vi "Generic command handler.vi"(8 "error in (no error)":errorcluster, 10 "Message in":refnum<class "GenericMessage.lvclass">, 11 "DAQMH121119OrcaFlash in":refnum<class "DAQOrcaFlash.lvclass">) -> (0 "error out":errorcluster, 2 "value":string, 3 "DAQMH121119OrcaFlash out":refnum<class "DAQOrcaFlash.lvclass">)   [LabVIEW 2012, in "DAQOrcaFlash.lvclass"]
doc: "The generic_command_handler processes the command 'generic'. Commands which are not part of the predefined list of commands fall under the 'generic' command for special activity."
uses:
  DAQOrcaFlash.lvclass
  <vilib>/Distrio/Murmex/GenericMessage/GenericMessage.lvclass
  <vilib>/Distrio/Murmex/Murmex/Murmex.lvclass
  <vilib>/Distrio/Murmex/ProceedMessage/ProceedMessage.lvclass
  DAQOrcaFlash.lvclass/DAQOrcaFlash.ctl
  <vilib>/Distrio/Murmex/Message/Message.lvclass
  <vilib>/Distrio/Murmex/ResetMessage/ResetMessage.lvclass
panel:
  # "This method is called when the GENERIC\ntrigger is sent. \n\nOverride this method when your component needs to\nrespond to this trigger. \n\nCall parent for proper implementation"
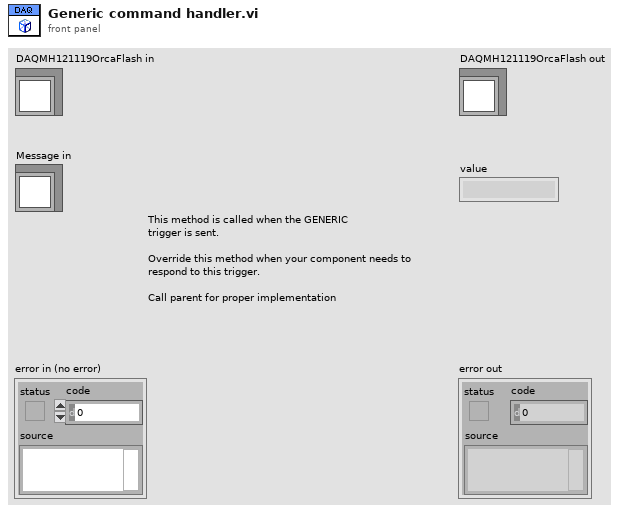
[diagram p1: front panel]
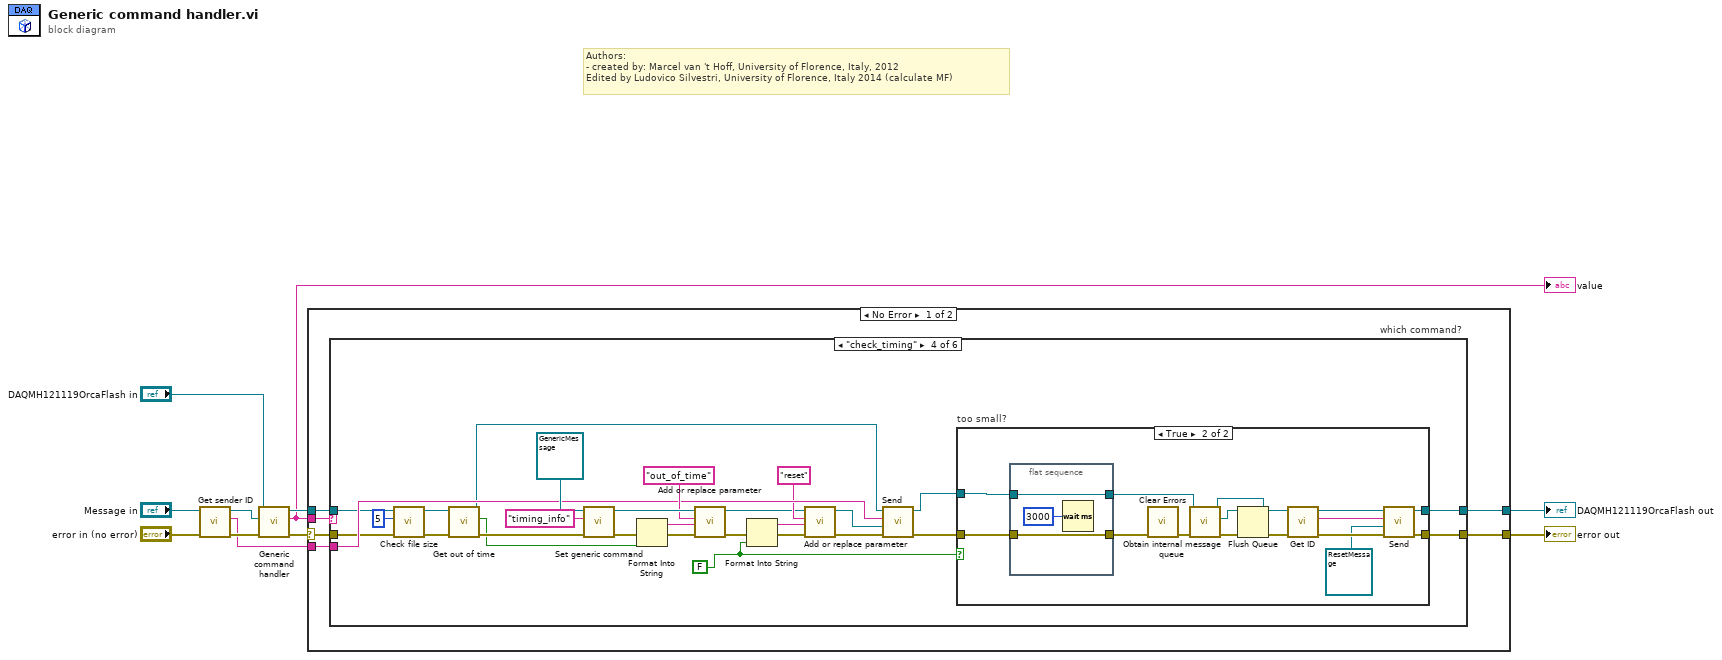
[diagram p0: block diagram]
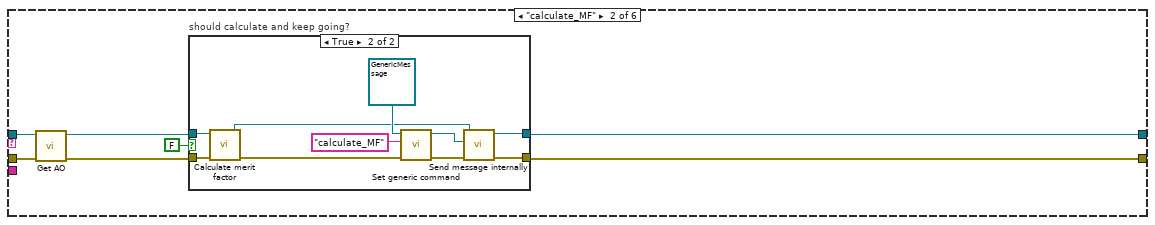
[diagram p3: hidden frame]
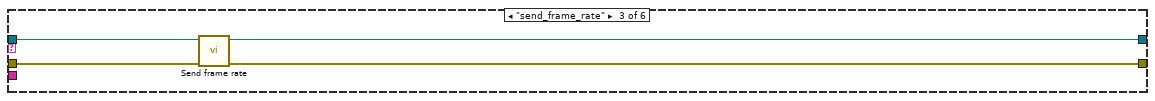
[diagram p5: hidden frame]
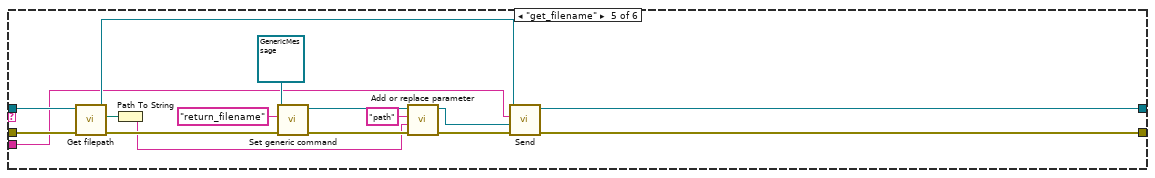
[diagram p7: hidden frame]
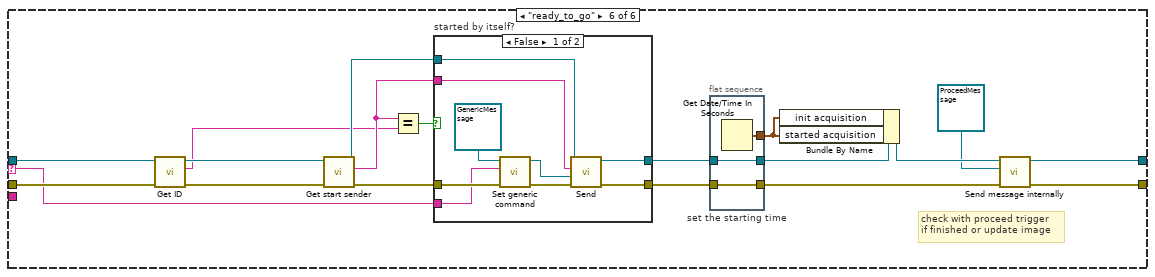
[diagram p8: hidden frame]
diagram:
  # "Authors: \n- created by: Marcel van 't Hoff, University of Florence, Italy, 2012\nEdited by Ludovico Silvestri, University of Florence, Italy 2014 (calculate MF)"
  n1 = call <vilib>:"Get sender ID.vi"("error in (no error)"="error in (no error)", "Message in"="Message in") -> ("error out"=w4:errorcluster, "sender"=w1:string, "Message out"=w2:refnum<class "GenericMessage.lvclass">)  [unwired: 7 in]
  n2 = call-parent "Generic command handler.vi"("error in (no error)"=w4, "Message in"=w2, "Murmex in"="DAQMH121119OrcaFlash in") -> ("error out"=w9:errorcluster, "value"=w5:string, "Murmex out"=w6:refnum<class "DAQOrcaFlash.lvclass">)  [unwired: 6 in]
  "value" <- w5
  n3 = case shown="No Error" w9 {
    selector: w9 -> [w16 w141]
    tunnel: [w15 w141] -> w8
    tunnel: [w14 w140] -> w7
    tunnel: w6 -> [w13 w140]
    tunnel: w5 -> [w17 _]
    tunnel: w1 -> [w12 _]
    frame No Error {
      n4 = case "which command?" shown="\"check_timing\"" w17 {
        selector: w17 -> [_ _ _ _ _ w123]
        tunnel: w16 -> [w19 w26 w42 w57 w105 w125]
        tunnel: w13 -> [w18 w25 w41 w59 w106 w120]
        tunnel: [w19 w22 w40 w44 w91 w110] -> w15
        tunnel: [w18 w21 w39 w45 w92 w108] -> w14
        tunnel: w12 -> [_ _ _ w63 w94 _]
        frame Default {
        }
        frame "calculate_MF" {
          n5 = call-dynamic "Get AO.vi"("error in (no error)"=w26, "DAQOrcaFlash in"=w25) -> ("error out"=w24:errorcluster, "DAQOrcaFlash out"=w23:refnum<class "DAQOrcaFlash.lvclass">)  [unwired: 7 in, 1 out]
          n6 = case "should calculate and keep going?" shown="True" FALSE {
            tunnel: w24 -> [w28 w38]
            tunnel: w23 -> [w27 w37]
            tunnel: [w28 w32] -> w22
            tunnel: [w27 w34] -> w21
            frame False {
            }
            frame True {
              n7 = call-dynamic "Calculate merit factor.vi"("error in (no error)"=w38, "DAQOrcaFlash in"=w37) -> ("error out"=w29:errorcluster, "DAQOrcaFlash out"=w30:refnum<class "DAQOrcaFlash.lvclass">)  [unwired: 8 in]
              n8 = call <vilib>:"Set generic command.vi"("error in (no error)"=w29, "generic command"="calculate_MF", "GenericMessage in"=refnum<class "GenericMessage.lvclass"> refnum ("GenericMessage")) -> ("error out"=w33:errorcluster, "GenericMessage out"=w31:refnum<class "GenericMessage.lvclass">)  [unwired: 7 in]
              n9 = call <vilib>:"Send message internally.vi"("error in (no error)"=w33, "Message"=w31, "Murmex in"=w30) -> ("error out"=w32:errorcluster, "Murmex out"=w34:refnum<class "DAQOrcaFlash.lvclass">)  [unwired: 7 in]
            }
          }
        }
        frame "send_frame_rate" {
          n10 = call-dynamic "Send frame rate.vi"("error in (no error)"=w42, "DAQOrcaFlash in"=w41) -> ("error out"=w40:errorcluster, "DAQOrcaFlash out"=w39:refnum<class "DAQOrcaFlash.lvclass">)  [unwired: 8 in]
        }
        frame "check_timing" {
          w43 = FALSE
          n11 = call-dynamic "Check file size.vi"("error in (no error)"=w57, "min size (KB)"=i64 5, "DAQOrcaFlash in"=w59) -> ("error out"=w56:errorcluster, "DAQOrcaFlash out"=w58:refnum<class "DAQOrcaFlash.lvclass">)  [unwired: 6 in, 1 out]
          n12 = call-dynamic "Get out of time.vi"("error in (no error)"=w56, "DAQOrcaFlash in"=w58) -> ("error out"=w62:errorcluster, "out of time?"=w60:bool, "DAQOrcaFlash out"=w61:refnum<class "DAQOrcaFlash.lvclass">)  [unwired: 7 in]
          n13 = call <vilib>:"Set generic command.vi"("error in (no error)"=w62, "generic command"="timing_info", "GenericMessage in"=refnum<class "GenericMessage.lvclass"> refnum ("Distrio Murmex 1.5:GenericMessage")) -> ("error out"=w66:errorcluster, "GenericMessage out"=w68:refnum<class "GenericMessage.lvclass">)  [unwired: 7 in]
          n14 = Format Into String(error in=w66, w60) -> (resulting string=w64:string, error out=w65:errorcluster)  [unwired: 2 in]
          n15 = call <vilib>:"Add or replace parameter.vi"("error in (no error)"=w65, "value"=w64, "name"="out_of_time", "Message in"=w68) -> ("error out"=w51:errorcluster, "Message out"=w49:refnum<class "GenericMessage.lvclass">)  [unwired: 6 in]
          n16 = Format Into String(error in=w51, w43) -> (resulting string=w52:string, error out=w53:errorcluster)  [unwired: 2 in]
          n17 = call <vilib>:"Add or replace parameter.vi"("error in (no error)"=w53, "value"=w52, "name"="reset", "Message in"=w49) -> ("error out"=w50:errorcluster, "Message out"=w48:refnum<class "GenericMessage.lvclass">)  [unwired: 6 in]
          n18 = call <vilib>:"Send.vi"("error in (no error)"=w50, "Message"=w48, "recipient"=w63, "Murmex in"=w61) -> ("error out"=w46:errorcluster, "Murmex out"=w47:refnum<class "DAQOrcaFlash.lvclass">)  [unwired: 6 in]
          n19 = case "too small?" shown="True" w43 {
            tunnel: w46 -> [w72 w83]
            tunnel: w47 -> [w71 w81]
            tunnel: [w72 w79] -> w44
            tunnel: [w71 w75] -> w45
            frame False {
            }
            frame True {
              n20 = flat-sequence {
                tunnel: [w90] -> w84
                tunnel: w83 -> [w90]
                tunnel: [w89] -> w82
                tunnel: w81 -> [w89]
                frame #0 {
                  n21 = Wait (ms)(milliseconds to wait=u32 3000) -> ()  [unwired: 1 out]
                }
              }
              n22 = call <vilib>:"Clear Errors.vi"("error in (no error)"=w84) -> ("error out"=w87:errorcluster)  [unwired: 6 in]
              n23 = call <vilib>:"Obtain internal message queue.vi"("error in (no error)"=w87, "Murmex in"=w82) -> ("error out"=w85:errorcluster, "internal message queue"=w86:refnum<queue>, "Murmex out"=w77:refnum<class "DAQOrcaFlash.lvclass">)  [unwired: 7 in]
              n24 = Flush Queue(queue=w86, error in (no error)=w85) -> (error out=w78:errorcluster)  [unwired: 2 out]
              n25 = call <vilib>:"Get ID.vi"("error in (no error)"=w78, "Murmex in"=w77) -> ("error out"=w80:errorcluster, "component id"=w74:string, "Murmex out"=w76:refnum<class "DAQOrcaFlash.lvclass">)  [unwired: 7 in]
              n26 = call <vilib>:"Send.vi"("error in (no error)"=w80, "Message"=refnum<class "ResetMessage.lvclass"> refnum ("Message in"), "recipient"=w74, "Murmex in"=w76) -> ("error out"=w79:errorcluster, "Murmex out"=w75:refnum<class "DAQOrcaFlash.lvclass">)  [unwired: 6 in]
            }
          }
        }
        frame "get_filename" {
          n27 = call "Get filepath.vi"("error in (no error)"=w105, "DAQOrcaFlash in"=w106) -> ("error out"=w102:errorcluster, "full storage path"=w98:path, "DAQOrcaFlash out"=w95:refnum<class "DAQOrcaFlash.lvclass">)  [unwired: 7 in]
          n28 = Path To String(path=w98) -> (string=w97:string)
          n29 = call <vilib>:"Set generic command.vi"("error in (no error)"=w102, "generic command"="return_filename", "GenericMessage in"=refnum<class "GenericMessage.lvclass"> refnum ("Message in")) -> ("error out"=w101:errorcluster, "GenericMessage out"=w100:refnum<class "GenericMessage.lvclass">)  [unwired: 7 in]
          n30 = call <vilib>:"Add or replace parameter.vi"("error in (no error)"=w101, "value"=w97, "name"="path", "Message in"=w100) -> ("error out"=w96:errorcluster, "Message out"=w93:refnum<class "GenericMessage.lvclass">)  [unwired: 6 in]
          n31 = call <vilib>:"Send.vi"("error in (no error)"=w96, "Message"=w93, "recipient"=w94, "Murmex in"=w95) -> ("error out"=w91:errorcluster, "Murmex out"=w92:refnum<class "DAQOrcaFlash.lvclass">)  [unwired: 6 in]
        }
        frame "ready_to_go" {
          # "check with proceed trigger\nif finished or update image"
          n32 = call <vilib>:"Get ID.vi"("error in (no error)"=w125, "Murmex in"=w120) -> ("error out"=w121:errorcluster, "component id"=w116:string, "Murmex out"=w119:refnum<class "DAQOrcaFlash.lvclass">)  [unwired: 7 in]
          n33 = call-dynamic "Get start sender.vi"("error in (no error)"=w121, "DAQOrcaFlash in"=w119) -> ("error out"=w124:errorcluster, "start sender"=w117:string, "DAQOrcaFlash out"=w122:refnum<class "DAQOrcaFlash.lvclass">)  [unwired: 7 in]
          n34 = Equal?(x=w117, y=w116) -> (x = y?=w118:bool)
          n35 = case "started by itself?" shown="False" w118 {
            tunnel: w124 -> [w134 w138]
            tunnel: w123 -> [w133 _]
            tunnel: w122 -> [w132 w139]
            tunnel: w117 -> [w131 _]
            tunnel: [w130 w139] -> w111
            tunnel: [w129 w138] -> w113
            frame False {
              n36 = call <vilib>:"Set generic command.vi"("error in (no error)"=w134, "generic command"=w133, "GenericMessage in"=refnum<class "GenericMessage.lvclass"> refnum ("Distrio Murmex 1.2:GenericMessage")) -> ("error out"=w137:errorcluster, "GenericMessage out"=w135:refnum<class "GenericMessage.lvclass">)  [unwired: 7 in]
              n37 = call <vilib>:"Send.vi"("error in (no error)"=w137, "Message"=w135, "recipient"=w131, "Murmex in"=w132) -> ("error out"=w129:errorcluster, "Murmex out"=w130:refnum<class "DAQOrcaFlash.lvclass">)  [unwired: 6 in]
            }
            frame True {
            }
          }
          n38 = flat-sequence "set the starting time" {
            tunnel: [w128] -> w115
            tunnel: w111 -> [w128]
            tunnel: w113 -> [w127]
            tunnel: [w127] -> w112
            tunnel: [w126] -> w114
            frame #0 {
              n39 = Get Date/Time In Seconds() -> (seconds since 1Jan1904=w126:timestamp)
            }
          }
          n40 = Bundle By Name(cluster=w115, "init acquisition"=w114, "started acquisition"=w114) -> (w109:refnum<class "DAQOrcaFlash.lvclass">)
          n41 = call <vilib>:"Send message internally.vi"("error in (no error)"=w112, "Message"=refnum<class "ProceedMessage.lvclass"> refnum ("ProceedMessage"), "Murmex in"=w109) -> ("error out"=w110:errorcluster, "Murmex out"=w108:refnum<class "DAQOrcaFlash.lvclass">)  [unwired: 7 in]
        }
      }
    }
    frame Error {
    }
  }
  "error out" <- w8
  "DAQMH121119OrcaFlash out" <- w7
